vi "TagData.vi"(1 "Data":u32 format="%x", 2 "Tag":u8 format="%x") -> (0 "Data 2":u32 format="%x")   [LabVIEW 2014]
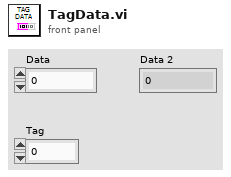
[diagram p1: front panel]
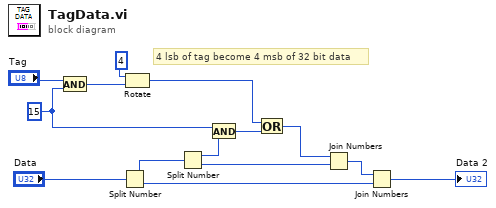
[diagram p0: block diagram]
diagram:
  w4 = u8 15 ("y")
  # "4 lsb of tag become 4 msb of 32 bit data"
  n1 = And(x="Tag", y=w4) -> (x .and. y?=w7:u8)
  n2 = Split Number(x="Data") -> (hi(x)=w13:u16, lo(x)=w12:u16)
  n3 = Rotate(1:w7, 2:u8 4 ("y")) -> (0:w1:u8)
  n4 = Split Number(x=w13) -> (hi(x)=w5:u8, lo(x)=w11:u8)
  n5 = And(x=w4, y=w5) -> (x .and. y?=w3:u8)
  n6 = Or(x=w1, y=w3) -> (x .or. y?=w2:u8)
  n7 = Join Numbers(hi=w2, lo=w11) -> ((hi.lo)=w10:u16)
  n8 = Join Numbers(hi=w10, lo=w12) -> ((hi.lo)=→"Data 2":u32)
